vi "Magna Interface Loop.vi"(1 "Magna IO Loop ID":u16, 11 "error in (no error)":errorcluster) -> ()   [LabVIEW 2011]
uses:
  Magna Commands.ctl
  Magna Configuration Values Set.ctl
  PCP interface/PSU Type.ctl
  Application Structure/Options/Action GFV Settings.ctl
  Magna PSU/Operating Modes Enum.ctl
  PCP interface/PCP Commands.ctl
  <vilib>/Instr/_visa.llb/VISA Flush IO Buffer Mask.ctl
  emi Lib/System 01/0 - General/App/Loop control 2/Private/_emi_ SMLoop start condition.vi
  emi Lib/System 01/0 - General/App/Loop control 2/Private/_emi_ SMLoop Error Check.vi
  emi Lib/Basic/0 - General/Error/emi_Is Error.vi
  emi Lib/System 01/0 - General/App/Loop control 2/Private/_emi_SMLoop Register new.vi
  emi Lib/System 01/0 - General/S&E reporting/emi_Send S&E Error message.vi
  emi Lib/Basic/0 - General/Error/emi_ Is Error state.vi
  emi Lib/System 01/0 - General/emi_Read System ID.vi
  emi Lib/System 01/0 - General/App/Loop control/Private/_emi_GFV Loop Linking.vi
  emi Lib/System 01/0 - General/App/Loop control/Private/_emi_GFV Loop Enable.vi
  emi Lib/System 01/0 - General/App/Loop control 2/Private/_emi_ SMLoop Restart.vi
  emi Lib/System 01/0 - General/App/Private/_emi_GFV App Close.vi
  emi Lib/System 01/0 - General/App/Loop control 2/Private/_emi_ SMLoop Restart Counter.vi
  emi Lib/System 01/0 - General/App/Loop control/Private/_emi_GFV Loop Running.vi
  emi Lib/System 01/0 - General/Private/_emi_GFV System ID.vi
  emi Lib/System 01/0 - General/S&E reporting/Private/_emi_S&E Q Generator.vi
  emi Lib/System 01/0 - General/App/Loop control/Private/_emi_GFV stop a loop so it can reset.vi
  Magna PSU.lvlib
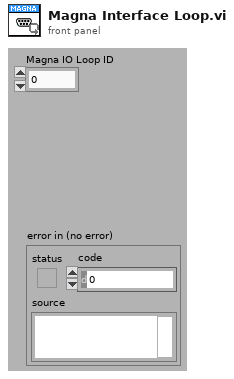
[diagram p1: front panel]
types:
  T1 = typedef "Magna Commands.ctl" = enum16{"Read Inputs", "HV ON", "HV OFF", "Set Resistance", "Set Head Voltage SP"}
  T2 = typedef "PSU Type.ctl" = enum16{"Unipower", "Magna 8.3A", "Magna 12A", "None"}
  T3 = typedef "Action GFV Settings.ctl" = enum16{"Init", "Get From INI", "Put In INI", "Get Settings", "Get Update Index", "Set Setting"}
  T4 = typedef "Magna PSU.lvlib/Operating Modes Enum.ctl" = enum16{"ROTARY", "KEYPAD", "EXT PGM", "REMOTE"}
  T5 = typedef "PCP Commands.ctl" = enum16{"do not use HE - Help", "RDd - Most used inputs", "RA - All analog inputs", "RE n Reset DO n", "SE n Set DO n", "RP - Get digital inputs", "VA d Set AO A  Motor Volt", "VB d Set AO B  Cable Resistance", "VEr - Get Version", "DYp - Depth counter", "DR - Reset Depth Counter", "DS n Set Depth options(0-3)", "do not use ME - Manual mode enabled", "MD - Manual mode disabled", "ID - Get ID(2001)", "TS - Get Timestamp", "TO d(s)  Set timeout", "do not use LO n Start Loop Mode(1,2)", "AL n RD&LO variation", "ST - Stop Loop Mode"}
  T6 = typedef "_emi_ SMLoop sates.ctl" = enum16{"Init", "Standby", "Start", "Normal Operation", "Stop", "Error Handling", "End", "Post"}
  T7 = typedef "Magna Configuration Values Set.ctl" = cluster{"Cable Resistance":dbl, "Voltage SP":dbl, "Over Voltage Protection":dbl, "Over Current Protection":dbl, "Voltage Rating":dbl, "Current Rating":dbl}
  T8 = cluster{"Placeholder":bool, "queue out":refnum<queue>, "VISA name":refnum<visa-resource-name>, "Configuration Values":T7}
  T9 = typedef "Options  All pages and custom.ctl" = cluster{"P 1 (App)":T10, "P 2":T11, "P 3":T12, "P 4":T14, "P 5":T19, "P 6 (Err)":T20, "P 7 (Expert)":T21, "P 8 (Depth)":T23, "C 1":T24, "C 2":T25}
  T10 = typedef "Options Page 1 (App).ctl" = cluster{"Result files":path, "PCP Interface":string, "Tractor/Stroker Interface":string, "Tractor Interface":string, "Modem Status Interface":string, "Audible Alarm":bool, "Force alarm on Technical":bool, "Force alarm on HH":bool, "Force alarm on LL":bool, "Force alarm on H":bool, "Force alarm on L":bool}
  T11 = typedef "Options Page 2.ctl" = cluster{"Solenoid & Relay latching time":u16, "Tractor relay 1":dbl, "Tractor relay 2":dbl, "Tractor Solenoid limit":dbl}
  T12 = typedef "Options Page 3.ctl" = cluster{"Min resistance":dbl, "Max resistance":dbl, "Head voltage range":T13, "Max voltage jump":dbl, "Maximum resistance change":dbl, "Start Telemetry Voltage":dbl, "Start Telemetry Timeout":dbl, "Start Motor Voltage":dbl, "Stop Motor Voltage":dbl, "Pass Mode Warning Voltage":dbl, "Relay Switch Voltage":dbl, "Relay Status Loss Voltage":dbl, "Samples to average":i32, "PSU type DO NOT USE":T2, "Magna OVP":dbl, "Magna Current Limit":dbl}
  T13 = typedef "PCP type List.ctl" = enum16{"0 - 350V", "0 - 450V", "0 - 600V"}
  T14 = typedef "Options Page 4.ctl" = cluster{"Solenoid & Relay latching time":u16, "Stroker relay 1":dbl, "Stroker Relay 2":dbl, "Stroker Solenoid limit":dbl, "Force det.":T15, "Stroke force lim.":dbl, "Anchor Enabled Pressure":dbl, "Tacometer puls":dbl, "Default anchor behavior":T16, "Default stroker behavior":T17, "Default stroker force limit (tonne)":dbl, "Slips Size":T18}
  T15 = typedef "Stroke force selector.ctl" = enum16{"Stroke in = node 1", "Strok out = node 1"}
  T16 = typedef "Default anchor behavior.ctl" = enum16{"Do nothing", "Set Anchor", "Release Anchor"}
  T17 = typedef "Default stroker behavior.ctl" = enum16{"Do nothing", "Stop", "Go Out", "Go In"}
  T18 = typedef "Slips Type Radio.ctl" = enum32{"No Selection", "338 MRS", "3,9 MRS"}
  T19 = typedef "Options Page 5.ctl" = cluster{"Solenoid & Relay latching time":u16, "Driller relay 1":dbl, "Driller Relay 2":dbl, "Driller  Solenoid limit":dbl}
  T20 = typedef "Options Page 6 (Err).ctl" = cluster{"Error and event files":path}
  T21 = typedef "Options Page 7 (Expert).ctl" = cluster{"Show Debug":bool, "Log debug messages":bool, "Additional debug messages":bool, "Start Beagle with Simulator data":bool, "Workshop mode":bool, "Modem baud":u16, "enumCANCOM":bool, "Modem sim":T22, "Telemetry Timeout Disable":i32, "Buffer size":i32, "Upd regular data":bool, "Cable comp":cluster{"VMOD1 Voltage(V)":dbl, "VMOD2 Voltage(V)":dbl}}
  T22 = typedef "Modem simulation setup.ctl" = cluster{"Modem dealay sim":bool, "Sim baud Tx":u16, "Bit Error fraction Tx":dbl, "Sim baud Rx":u16, "Bit Error fraction Rx":dbl}
  T23 = typedef "Options Page 8 (Depth).ctl" = cluster{"Winch Spool Circumference":dbl, "Winch Pulses per Revolution":dbl, "Current Depth":dbl}
  T24 = typedef "Options Custom 1.ctl" = cluster{"Depth Updated":bool, "Depth Offset":dbl}
  T25 = typedef "Options Custom 2.ctl" = cluster{"Placeholder":bool}
  T26 = typedef "Magna Command Definer.ctl" = cluster{"Action":T1, "n(0)":i32, "d(0.0)":dbl}
  T27 = typedef "RDd return.ctl" = cluster{"AI":T28, "Depth counter(Raw)":i32, "General Ratemeter":dbl, "Digital ports":T29}
  T28 = typedef "RA return Analog I.ctl" = cluster{"HVPSU voltage output (AI 1)":dbl, "HVPSU current output (AI 2)":dbl, "PCP Motor voltage, head voltage (AI 3)":dbl, "PCP Cable resistance (AI 4)":dbl, "Cable tension (AI 5)":dbl, "CCL (AI 6)":dbl}
  T29 = typedef "RP return digital IO.ctl" = cluster{"DO -  HVPSU HV Off":bool, "DO -  HVPSU HV On":bool, "DI -  Unused 1":bool, "DO -  Local(T) / PC(F) mode":bool, "DI - Unused 2":bool, "DI - HVPSU HV On(T)":bool, "DI - PCP Local control(T)":bool, "DI - HVPSU On(T)":bool}
  T30 = typedef "VISA Flush IO Buffer Mask.ctl" = u16
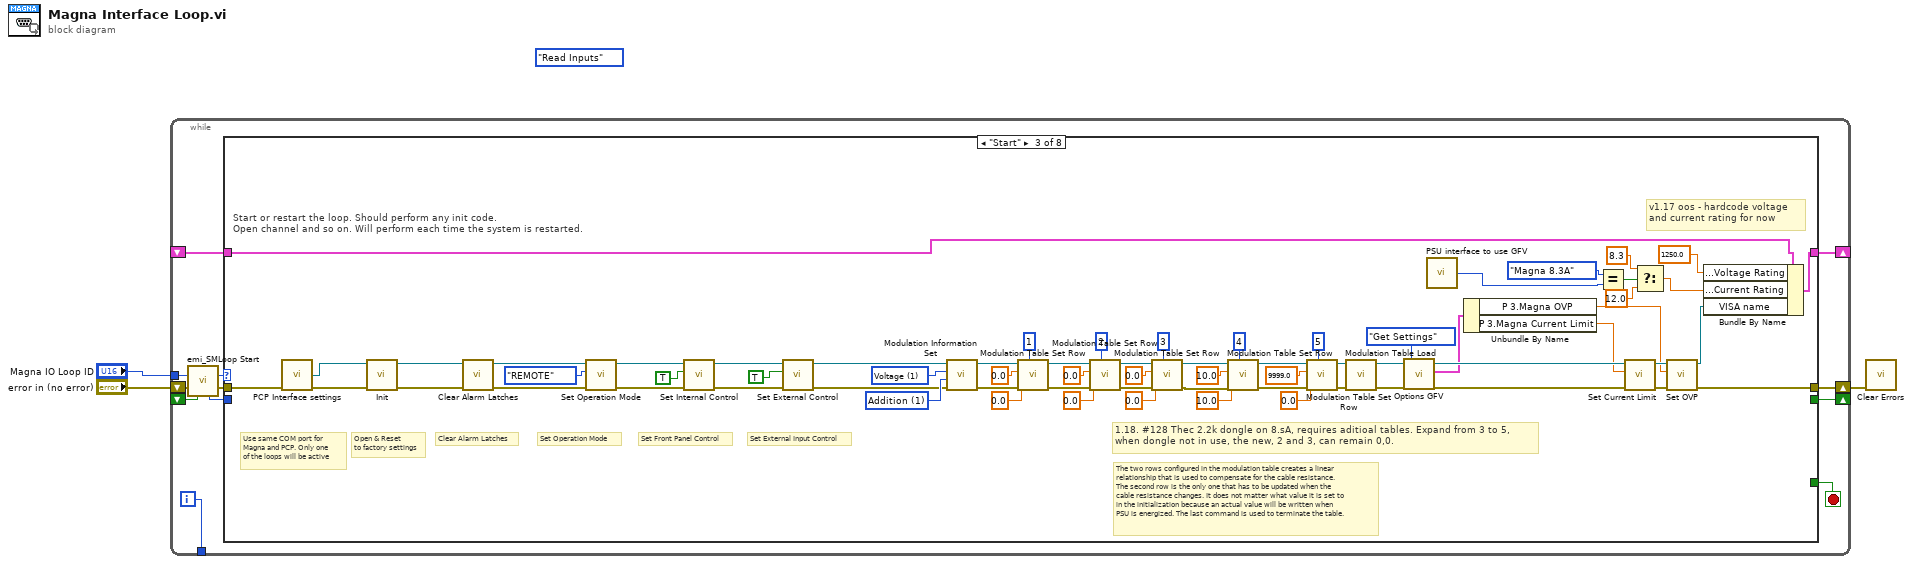
[diagram p0: block diagram]
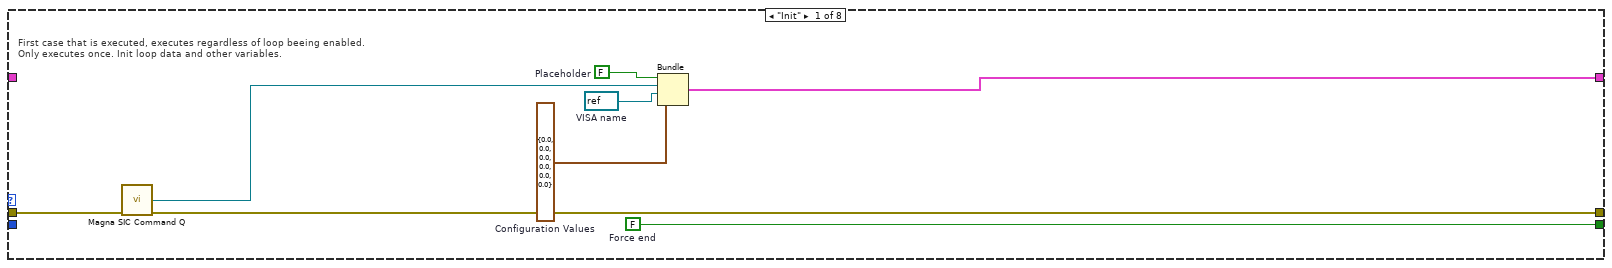
[diagram p2: hidden frame]
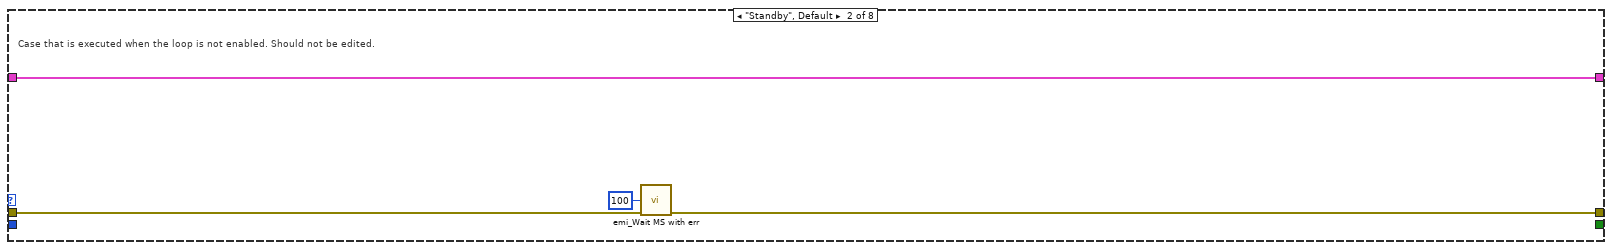
[diagram p3: hidden frame]
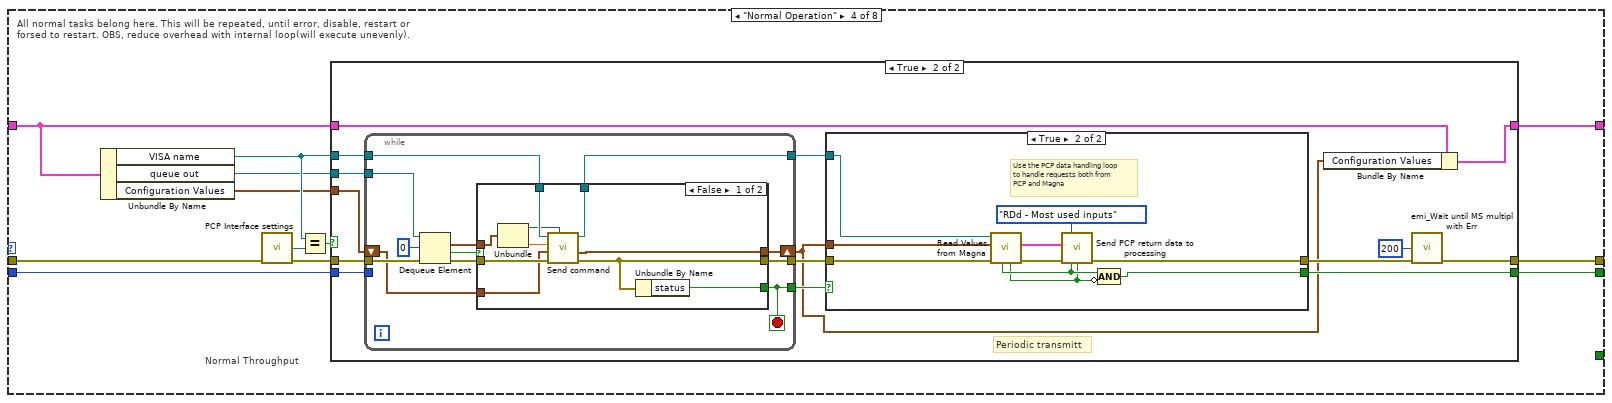
[diagram p4: hidden frame]
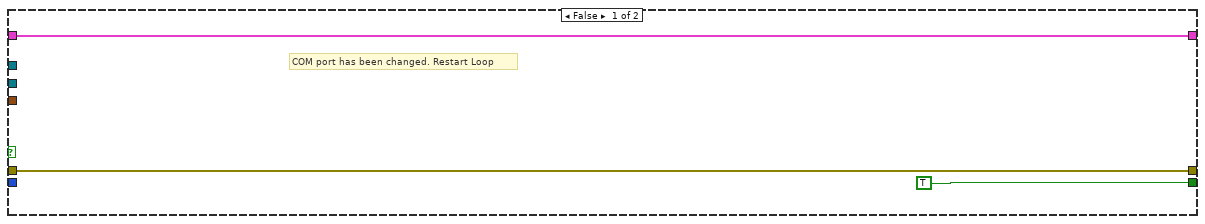
[diagram p5: hidden frame]
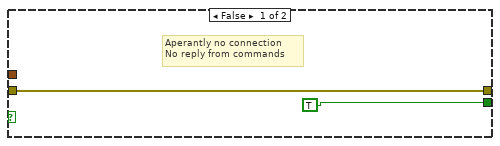
[diagram p6: hidden frame]
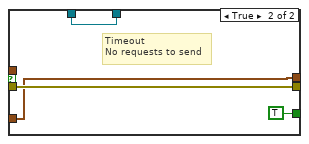
[diagram p7: hidden frame]
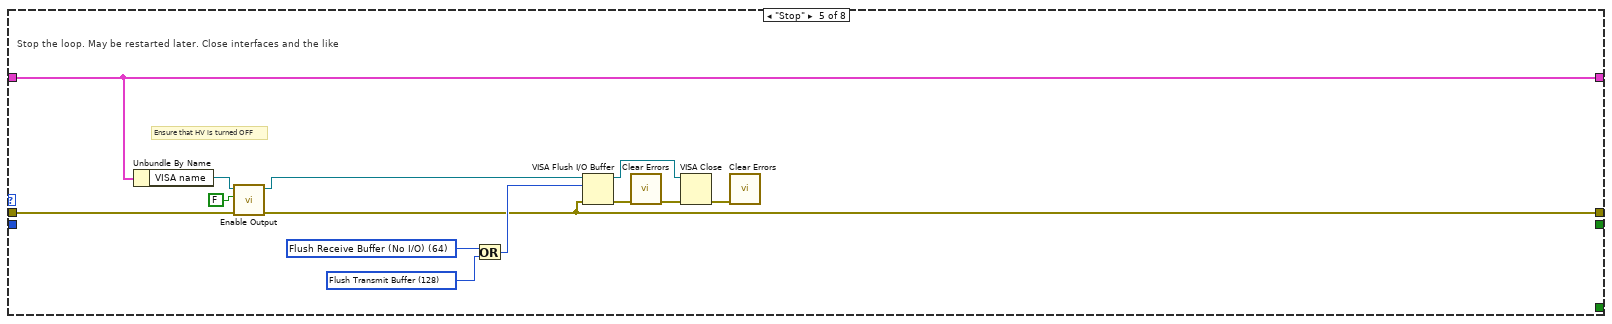
[diagram p8: hidden frame]
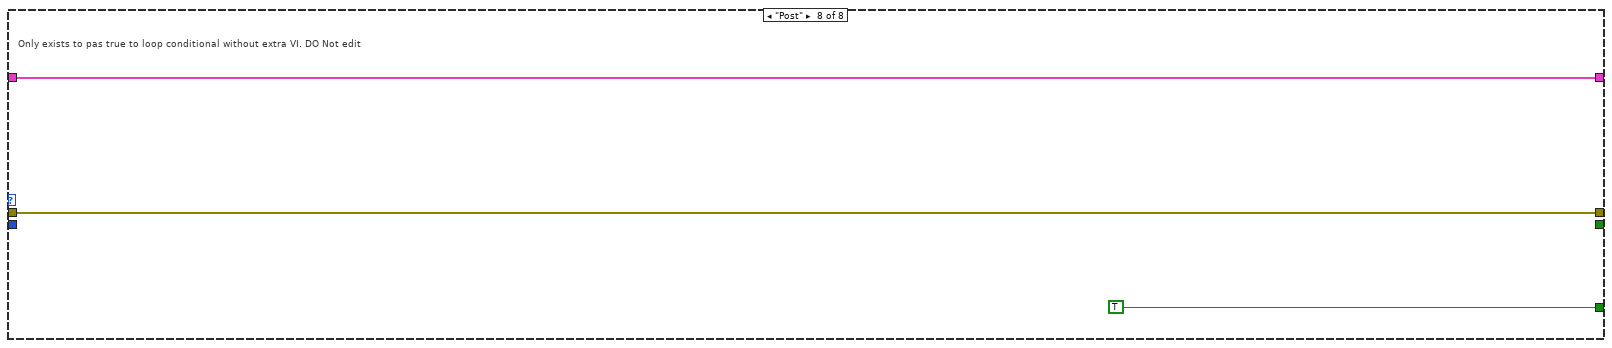
[diagram p11: hidden frame]
diagram:
  (unwired) Magna_Commands."Read Inputs" ("Action")
  n1 = while {
    shift-right: [w15] -> _
    shift-left: _ -> [w11]
    shift-right: [w13] -> w1
    shift-left: "error in (no error)" -> [w9]
    tunnel: [w12] -> _
    shift-right: [w10] -> _
    shift-left: _ -> [w5]
    tunnel: "Magna IO Loop ID" -> [w6]
    i -> [w12]
    stop <- w14 stop-if-true
    n2 = call "emi_SMLoop Start.vi"("Loop ID"=w6, "error in (no error)"=w9, "Force Stop(F)"=w5) -> ("Loop command"=w7:T6, "error out"=w8:errorcluster, "Loop ID out"=w4:i32)  [unwired: 10 in]
    n3 = case shown="\"Start\"" w7 {
      tunnel: [w21 w24 w91 w102 w172 w175 w176 w179] -> w15
      tunnel: [_ _ _ _ _ _ _ TRUE] -> w14
      tunnel: w8 -> [w19 w26 w92 w104 w164 w174 w177 w180]
      tunnel: [w18 w25 w55 w103 w163 w174 w177 w180] -> w13
      tunnel: w11 -> [_ w24 w43 w101 w172 w175 w176 w179]
      tunnel: [w22 _ _ w100 _ _ _ _] -> w10
      tunnel: w4 -> [_ _ _ w99 _ _ _ _]
      frame "Init" {
        w16 = T7 {"Cable Resistance"=0.0, "Voltage SP"=0.0, "Over Voltage Protection"=0.0, "Over Current Protection"=0.0, "Voltage Rating"=0.0, "Current Rating"=0.0}  # Configuration Values
        w20 = refnum<visa-resource-name> refnum  # VISA name
        w22 = FALSE  # Force end
        w23 = FALSE  # Placeholder
        # "First case that is executed, executes regardless of loop beeing enabled.\nOnly executes once. Init loop data and other variables."
        n4 = call "Magna SIC Command Q.vi"("error in (no error)"=w19) -> ("queue out"=w17:refnum<queue>, "error out"=w18:errorcluster)  [unwired: 13 in]
        n5 = Bundle("Placeholder"=w23, "queue out"=w17, "VISA name"=w20, "Configuration Values"=w16) -> (w21:T8)  [unwired: 1 in]
      }
      frame "Standby", Default {
        # "Case that is executed when the loop is not enabled. Should not be edited."
        n6 = call "emi_Wait MS with err.vi"("milliseconds to wait(0)"=u32 100, "error in (no error)"=w26) -> ("error out"=w25:errorcluster)  [unwired: 13 in]
      }
      frame "Start" {
        w77 = u16 1 items=["Multiplication", "Addition"] ("Modulation Type")
        w54 = i8 1 items=["None", "Voltage", "Current"] ("Select Output to Modulate")
        # "1.18. #128 Thec 2.2k dongle on 8.sA, requires aditioal tables. Expand from 3 to 5, \nwhen dongle not in use, the new, 2 and 3, can remain 0,0."
        # "v1.17 oos - hardcode voltage \nand current rating for now"
        # "The two rows configured in the modulation table creates a linear \nrelationship that is used to compensate for the cable resistance. \nThe second row is the only one that has to be updated when the \ncable resistance changes. It does not matter what value it is set to \nin the initialization because an actual value will be written when \nPSU is energized. The last command is used to terminate the table."
        # "Set Operation Mode"
        # "Set External Input Control"
        # "Set Front Panel Control"
        # "Clear Alarm Latches"
        # "Open & Reset\nto factory settings"
        # "Use same COM port for\nMagna and PCP. Only one\nof the loops will be active"
        # "Start or restart the loop. Should perform any init code. \nOpen channel and so on. Will perform each time the system is restarted."
        n7 = call "PCP Interface settings.vi"("error in (no error)"=w92) -> ("PCP VISA  name  out"=w90:refnum<visa-resource-name>, "error out"=w89:errorcluster)  [unwired: 13 in]
        n8 = call "Init.vi"("error in (no error)"=w89, "VISA resource name"=w90) -> ("error out"=w87:errorcluster, "VISA resource name out"=w88:refnum<visa-resource-name>)  [unwired: 8 in]
        n9 = call "Clear Alarm Latches.vi"("error in (no error)"=w87, "VISA Refnum in"=w88) -> ("error out"=w85:errorcluster, "VISA Refnum out"=w86:refnum<visa-resource-name>)  [unwired: 8 in]
        n10 = call "Set Operation Mode.vi"("error in (no error)"=w85, "Operating Modes"=Operating_Modes_Enum."REMOTE", "VISA session"=w86) -> ("error out"=w81:errorcluster, "dup VISA session"=w82:refnum<visa-resource-name>)  [unwired: 7 in]
        n11 = call "Set Internal Control.vi"("error in (no error)"=w81, "Internal Control"=TRUE, "VISA session"=w82) -> ("error out"=w79:errorcluster, "dup VISA session"=w80:refnum<visa-resource-name>)  [unwired: 7 in]
        n12 = call "Set External Control.vi"("error in (no error)"=w79, "External Control"=TRUE ("Internal Control"), "VISA session"=w80) -> ("error out"=w75:errorcluster, "dup VISA session"=w76:refnum<visa-resource-name>)  [unwired: 7 in]
        n13 = call "Modulation Information Set.vi"("error in (no error)"=w75, "Modulation Type"=w77, "Select Output to Modulate"=w54, "VISA session"=w76) -> ("error out"=w72:errorcluster, "dup VISA session"=w73:refnum<visa-resource-name>)  [unwired: 6 in]
        n14 = call "Modulation Table Set Row.vi"("Row"=i8 1, "error in (no error)"=w72, "Modulation Factor"=0.0, "Modulation Voltage"=0.0, "VISA session in"=w73) -> ("error out"=w34:errorcluster, "VISA session out"=w33:refnum<visa-resource-name>)  [unwired: 5 in]
        n15 = call "Modulation Table Set Row.vi"("Row"=i8 2, "error in (no error)"=w34, "Modulation Factor"=0.0, "Modulation Voltage"=0.0, "VISA session in"=w33) -> ("error out"=w32:errorcluster, "VISA session out"=w31:refnum<visa-resource-name>)  [unwired: 5 in]
        n16 = call "Modulation Table Set Row.vi"("Row"=i8 3, "error in (no error)"=w32, "Modulation Factor"=0.0, "Modulation Voltage"=0.0, "VISA session in"=w31) -> ("error out"=w29:errorcluster, "VISA session out"=w30:refnum<visa-resource-name>)  [unwired: 5 in]
        n17 = call "Modulation Table Set Row.vi"("Row"=i8 4, "error in (no error)"=w29, "Modulation Factor"=10.0, "Modulation Voltage"=10.0, "VISA session in"=w30) -> ("error out"=w62:errorcluster, "VISA session out"=w63:refnum<visa-resource-name>)  [unwired: 5 in]
        n18 = call "Modulation Table Set Row.vi"("Row"=i8 5, "error in (no error)"=w62, "Modulation Factor"=0.0, "Modulation Voltage"=9999.0, "VISA session in"=w63) -> ("error out"=w60:errorcluster, "VISA session out"=w61:refnum<visa-resource-name>)  [unwired: 5 in]
        n19 = call "Modulation Table Load.vi"("error in (no error)"=w60, "VISA session in"=w61) -> ("error out"=w52:errorcluster, "VISA session out"=w59:refnum<visa-resource-name>)  [unwired: 8 in]
        n20 = call "Options GFV.vi"("error in (no error)"=w52, "Action(Get Settings)"=Action_GFV_Settings."Get Settings") -> ("Options"=w50:T9, "error out"=w51:errorcluster)  [unwired: 15 in, 1 out]
        n21 = call "PSU interface to use GFV.vi"() -> ("PSU type  out"=w28:T2)  [unwired: 14 in, 1 out]
        n22 = Unbundle By Name(w50) -> ("P 3.Magna OVP"=w49:dbl, "P 3.Magna Current Limit"=w48:dbl)
        n23 = Equal?(x=PSU_Type."Magna 8.3A" ("P 3.PSU type"), y=w28) -> (x = y?=w45:bool)
        n24 = call "Set Current Limit.vi"("error in (no error)"=w51, "Set Current"=w48, "VISA session"=w59) -> ("error out"=w57:errorcluster, "dup VISA session"=w58:refnum<visa-resource-name>)  [unwired: 7 in]
        n25 = Select(t=8.3, s=w45, f=12.0) -> (s? t:f=w41:dbl)
        n26 = call "Set OVP.vi"("error in (no error)"=w57, "Set OVP"=w49, "VISA session"=w58) -> ("error out"=w55:errorcluster, "dup VISA session"=w56:refnum<visa-resource-name>)  [unwired: 7 in]
        n27 = Bundle By Name(cluster=w43, "Configuration Values.Voltage Rating"=1250.0, "Configuration Values.Current Rating"=w41, "VISA name"=w56) -> (w91:T8)
      }
      frame "Normal Operation" {
        # "Normal Throughput"
        # "All normal tasks belong here. This will be repeated, until error, disable, restart or\nforsed to restart. OBS, reduce overhead with internal loop(will execute unevenly)."
        n28 = Unbundle By Name(w101) -> ("VISA name"=w95:refnum<visa-resource-name>, "queue out"=w94:refnum<queue>, "Configuration Values"=w93:T7)
        n29 = call "PCP Interface settings.vi"("error in (no error)"=w104) -> ("PCP VISA  name  out"=w98:refnum<visa-resource-name>, "error out"=w96:errorcluster)  [unwired: 13 in]
        n30 = Equal?(x=w95, y=w98) -> (x = y?=w97:bool)
        n31 = case shown="True" w97 {
          tunnel: w96 -> [w106 w122]
          tunnel: [w105 w109] -> w102
          tunnel: w101 -> [w105 w110]
          tunnel: [TRUE ("Force End") w116] -> w100
          tunnel: [w106 w115] -> w103
          tunnel: w94 -> [_ w121]
          tunnel: w95 -> [_ w120]
          tunnel: w99 -> [_ w119]
          tunnel: w93 -> [_ w111]
          frame False {
            # "COM port has been changed. Restart Loop"
          }
          frame True {
            # "Periodic transmitt"
            n32 = while {
              tunnel: w122 -> [w145]
              tunnel: w121 -> [w144]
              tunnel: w120 -> [w141]
              tunnel: w119 -> [_]
              tunnel: [w140] -> w117
              tunnel: [w138] -> w118
              tunnel: [w137] -> w112
              shift-right: [w136] -> w108
              shift-left: w111 -> [w135]
              stop <- w137 stop-if-true
              n33 = Dequeue Element(queue=w144, timeout in ms (-1)=0, error in (no error)=w145) -> (element=w142:T26, timed out?=w139:bool, error out=w143:errorcluster)  [unwired: 1 out]
              n34 = case shown="False" w139 {
                tunnel: w143 -> [w154 w159]
                tunnel: [w150 w159] -> w138
                tunnel: w142 -> [w156 _]
                tunnel: w141 -> [w153 w160]
                tunnel: [w155 w160] -> w140
                tunnel: [w149 TRUE ("status")] -> w137
                tunnel: [w148 w157] -> w136
                tunnel: w135 -> [w147 w157]
                frame False {
                  n35 = Unbundle(w156) -> ("Action"=w152:T1, "d(0.0)"=w151:dbl)  [unwired: 1 out]
                  n36 = call "Send command.vi"("Action"=w152, "error in (no error)"=w154, "Set Values in"=w147, "d(0.0)"=w151, "VISA resource"=w153) -> ("error out"=w150:errorcluster, "Set Values"=w148:T7, "VISA resource out"=w155:refnum<visa-resource-name>)  [unwired: 4 in]
                  n37 = Unbundle By Name(w150) -> ("status"=w149:bool)
                }
                frame True {
                  # "Timeout\nNo requests to send"
                }
              }
            }
            n38 = case shown="True" w112 {
              tunnel: w118 -> [w124 w127]
              tunnel: [w124 w134] -> w114
              tunnel: w117 -> [_ w126]
              tunnel: [TRUE w132] -> w116
              tunnel: w108 -> [_ w125]
              frame False {
                # "Aperantly no connection\nNo reply from commands"
              }
              frame True {
                # "Use the PCP data handling loop\nto handle requests both from \nPCP and Magna"
                n39 = call "Read Values from Magna.vi"("error in (no error)"=w127, "Set Values in"=w125, "VISA session in"=w126) -> ("error out"=w131:errorcluster, "output cluster"=w130:T27, "Reply Expected"=w128:bool, "Reply Received"=w129:bool)  [unwired: 4 in, 1 out]
                n40 = call "Send PCP return data to processing.vi"("PCP Action"=PCP_Commands."RDd - Most used inputs" ("Action"), "Return Data"=w130, "error in"=w131, "Reply Received"=w129, "Reply Expected"=w128) -> ("error out"=w134:errorcluster)  [unwired: 10 in]
                n41 = Compound Arithmetic op=AND(w129, invert w128) -> (w132:bool)
              }
            }
            n42 = Bundle By Name(cluster=w110, "Configuration Values"=w108) -> (w109:T8)
            n43 = call "emi_Wait until MS multipl with Err.vi"("millisecond multiple(0)"=u32 200 ("milliseconds to wait(0)"), "error in (no error)"=w114) -> ("error out"=w115:errorcluster)  [unwired: 13 in]
          }
        }
      }
      frame "Stop" {
        w166 = T30 128 items=["Flush Receive Buffer"=16, "Write Transmit Buffer to Device"=32, "Flush Receive Buffer (No I/O)"=64, "Flush Transmit Buffer"=128] ("Mask")
        w168 = T30 64 items=["Flush Receive Buffer"=16, "Write Transmit Buffer to Device"=32, "Flush Receive Buffer (No I/O)"=64, "Flush Transmit Buffer"=128] ("Mask")
        # "Ensure that HV is turned OFF"
        # "Stop the loop. May be restarted later. Close interfaces and the like"
        n44 = Unbundle By Name(w172) -> ("VISA name"=w162:refnum<visa-resource-name>)
        n45 = call "Enable Output.vi"("error in (no error)"=w164, "Output Control"=FALSE, "VISA session"=w162) -> ("error out"=w163:errorcluster, "dup VISA session"=w161:refnum<visa-resource-name>)  [unwired: 7 in]
        n46 = Or(x=w168, y=w166) -> (x .or. y?=w167:T30)
        n47 = VISA Flush I/O Buffer(VISA resource name=w161, mask (16)=w167, error in (no error)=w163) -> (VISA resource name out=w169:refnum<visa-resource-name>, error out=w170:errorcluster)
        n48 = call <vilib>:"Clear Errors.vi"("error in (no error)"=w170) -> ("error out"=w171:errorcluster)  [unwired: 6 in]
        n49 = VISA Close(VISA resource name=w169, error in (no error)=w171) -> (error out=w173:errorcluster)
        n50 = call <vilib>:"Clear Errors.vi"("error in (no error)"=w173) -> ()  [unwired: 6 in, 1 out]
      }
      frame "Error Handling" {
        # "Loop automaticaly returns here after error is found. If error is cleared, \nLoop wil continue as normal(if was operative when error."
      }
      frame "End" {
        # "Only executes at application end has. Should performa any action the loop \nneeds to finnish. Executes only once."
      }
      frame "Post" {
        # "Only exists to pas true to loop conditional without extra VI. DO Not edit"
      }
    }
  }
  n51 = call <vilib>:"Clear Errors.vi"("error in (no error)"=w1) -> ()  [unwired: 6 in, 1 out]
